vi "GPIO Number.vi"(4 "GPIO in":refnum<class "GPIO.lvclass">) -> (7 "GPIO #":T1=-1)   [LabVIEW 2024, in "CTI.lvlib" / "GPIO.lvclass"]
uses:
  GPIO.lvclass
  GPIO Number.ctl
  GPIO.lvclass/GPIO.ctl
  CTI.lvlib
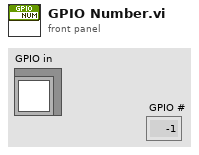
[diagram p1: front panel]
types:
  T1 = typedef "CTI.lvlib/GPIO Number.ctl" = i8
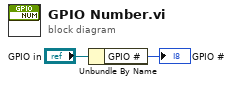
[diagram p0: block diagram]
diagram:
  n1 = Unbundle By Name("GPIO in") -> ("GPIO #"=→"GPIO #":T1)
